vi "DeQ Loop.vi"(10 "DVR Q":refnum<data-value>) -> ()   [LabVIEW 2021, in "DVR Qs.lvlib"]
uses:
  DVR Qs.lvlib
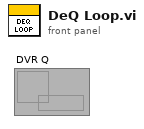
[diagram p1: front panel]
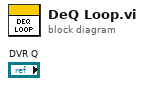
[diagram p0: block diagram]
diagram:
